vi "Write Events.vi"(8 "error in (no error)":errorcluster, 10 "Events":T1, 11 "In":refnum<class "base view.lvclass">) -> (0 "error out":errorcluster, 3 "Out":refnum<class "base view.lvclass">)   [LabVIEW 2022 SP3, in "base view.lvclass"]
uses:
  base view.lvclass
  Events.ctl
  base view.lvclass/base view.ctl
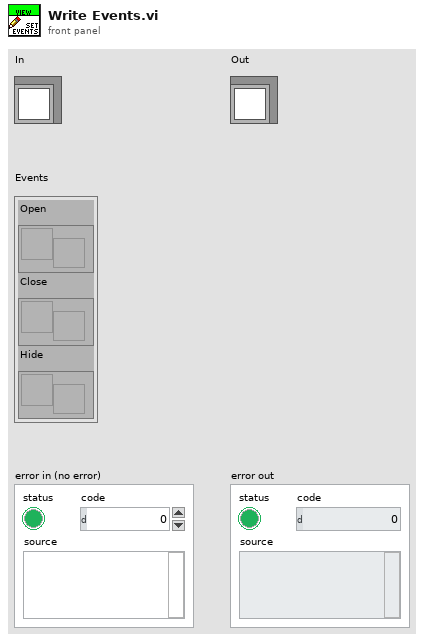
[diagram p1: front panel]
types:
  T1 = typedef "base view.lvclass/Events.ctl" = cluster{"Open":refnum<user-event>, "Close":refnum<user-event>, "Hide":refnum<user-event>}
  T2 = typedef "base view.lvclass/Data.ctl" = cluster{"View Refnum":refnum<vi>, "Wrapped View Refnum":refnum<vi>, "Events":T1, "event registration refnum":refnum<event-registration>}
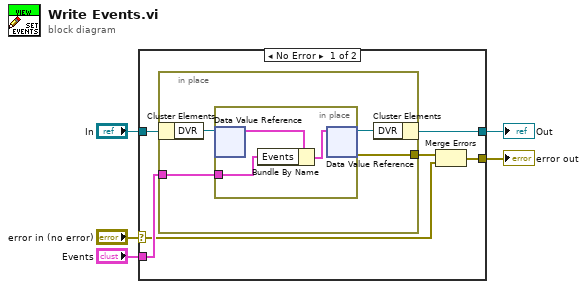
[diagram p0: block diagram]
diagram:
  n1 = case shown="No Error" "error in (no error)" {
    selector: "error in (no error)" -> [w6 w20]
    tunnel: [w7 w20] -> w4
    tunnel: [w11 w19] -> w3
    tunnel: "In" -> [w10 w19]
    tunnel: "Events" -> [w9 _]
    frame No Error {
      n2 = in-place {
        in-place-border: w9 -> [w13]
        in-place-border: [w12] -> w8
        n3 = in-place-cluster #1(w10) -> ("DVR"=w14:refnum<data-value>)
        n4 = in-place {
          in-place-border: w13 -> [w17]
          n5 = in-place-dvr #2(w14) -> (w16:T2)  [unwired: 1 out]
          n6 = Bundle By Name(cluster=w16, "Events"=w17) -> (w18:T2)
          n7 = in-place-dvr #2(w18) -> (w15:refnum<data-value>, w12:errorcluster)
        }
        n8 = in-place-cluster #1("DVR"=w15) -> (w11:refnum<class "base view.lvclass">)
      }
      n9 = Merge Errors(w8, w6) -> (w7:errorcluster)
    }
    frame Error {
    }
  }
  "Out" <- w3
  "error out" <- w4
